vi "Ping arp.vi"() -> (3 "IP Addresses Output":string[](array[string]))   [LabVIEW 2013]
panel:
  in  "Stop Button":bool
  out "standard output":string
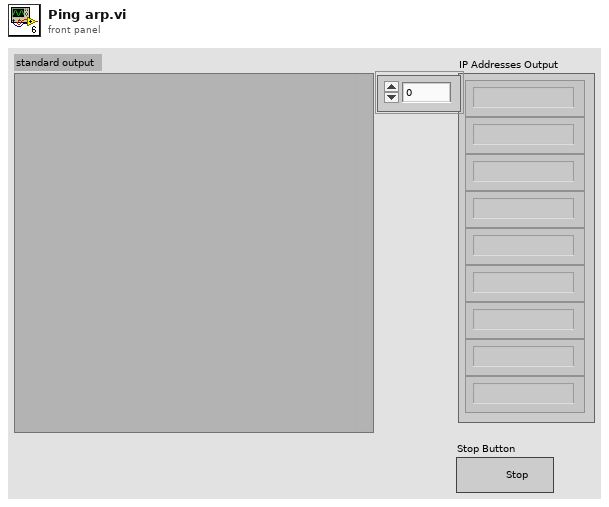
[diagram p1: front panel]
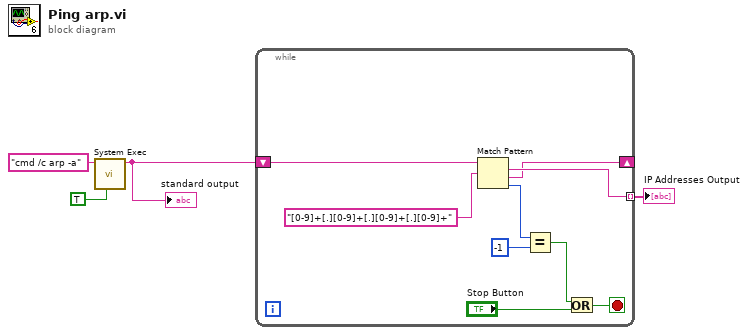
[diagram p0: block diagram]
diagram:
  n1 = call <vilib>:"System Exec.vi"("run minimized? (F)"=TRUE, "command line"="cmd /c arp -a") -> ("standard output"=w2:string)  [unwired: 6 in, 3 out]
  "standard output" <- w2
  n2 = while {
    tunnel: [w11] -> w1 mode=indexing
    shift-right: [w10] -> _
    shift-left: w2 -> [w12]
    stop <- w6 stop-if-true
    n3 = Match Pattern(string=w12, regular expression="[0-9]+[.][0-9]+[.][0-9]+[.][0-9]+") -> (match substring=w11:string, after substring=w10:string, offset past match=w8:i32)  [unwired: 1 in, 1 out]
    n4 = Equal?(x=w8, y=-1) -> (x = y?=w5:bool)
    n5 = Or(x=w5, y="Stop Button") -> (x .or. y?=w6:bool)
  }
  "IP Addresses Output" <- w1
